vi "Inject Fan Controller.vi"(8 "error in (no error)":errorcluster, 11 "iProcess Step Model in":refnum<class "iProcess Step Model.lvclass">) -> (0 "error out":errorcluster, 3 "iProcess Step Model out":refnum<class "iProcess Step Model.lvclass">)   [LabVIEW 2017, in "iProcess Step Model.lvclass"]
uses:
  D:/builds/Dynamic VI Handler/iProcess Step Model/iProcess Step Model.lvclass
panel:
  in  "String Control":string
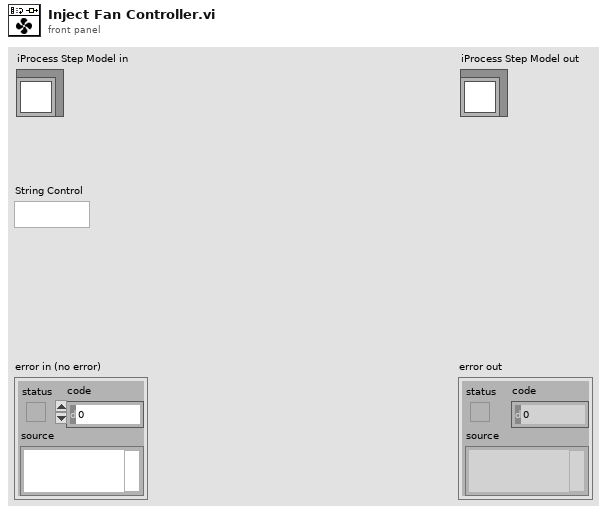
[diagram p1: front panel]
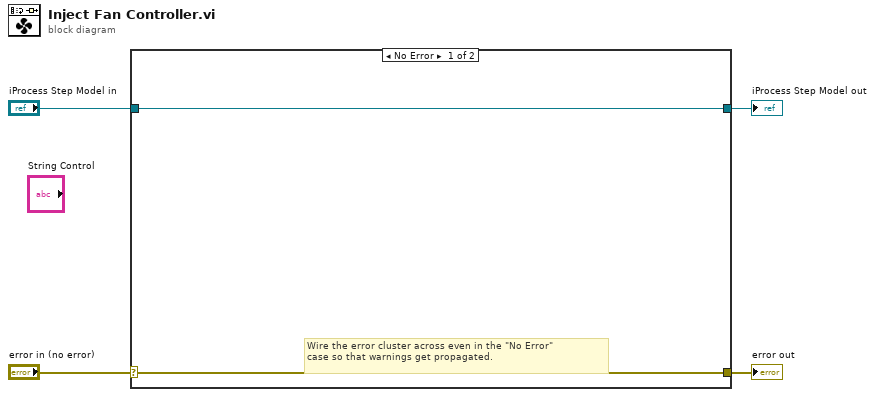
[diagram p0: block diagram]
diagram:
  n1 = case shown="No Error" "error in (no error)" {
    selector: "error in (no error)" -> [w5 w8]
    tunnel: [w5 w8] -> w3
    tunnel: [w6 w7] -> w1
    tunnel: "iProcess Step Model in" -> [w6 w7]
    frame No Error {
      # "Wire the error cluster across even in the \"No Error\"\ncase so that warnings get propagated."
    }
    frame Error {
    }
  }
  "error out" <- w3
  "iProcess Step Model out" <- w1
